vi "PQbuildConnectionString.vi"() -> ()   [LabVIEW 2019, in "libpqutility64.lvlib"]
doc: "Set up connection parameters, test the connectionstring and store it named into file. See PostgreSQL c-lib dokumentation for further information."
uses:
  libpqutility64.lvlib
  libpqlv/libpqlv.lvlib
  <vilib>/Utility/config.llb/NI_LVConfig.lvlib
  <vilib>/Utility/config.llb/Write Key (String).vi
panel:
  in  "Dateiname":string
  in  "Stopp":bool
  in  "Verbindungsname":string
  out "PQerrorMessage":string
  out "PQStatus":T1(ring)
  out "PQprotocolVersion":u32
  in  "Verbindung_testen":bool
  in  "Verbindung speichern":bool
  out "conninfo":string="\n"
  in  "requiressl":string
  in  "tty":string
  in  "options":string
  in  "connect_timeout":string
  in  "password":string
  in  "user":string
  in  "dbname":string
  in  "port":string
  in  "hostaddr":string
  in  "host":string
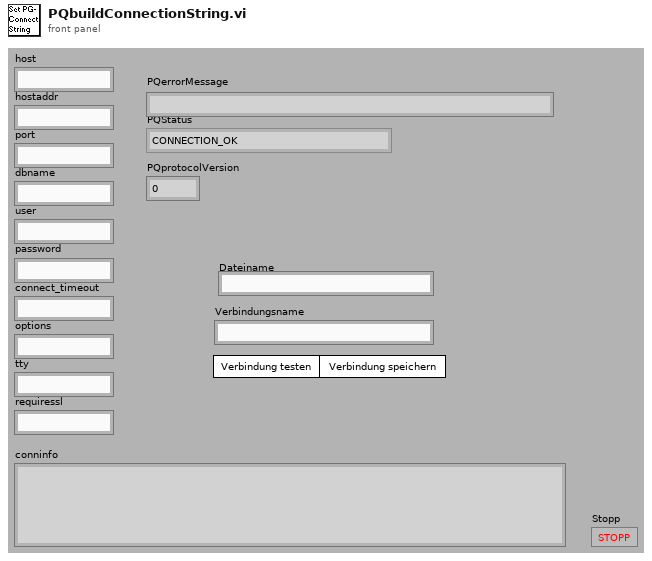
[diagram p1: front panel]
types:
  T1 = enum16{"CONNECTION_OK", "CONNECTION_BAD", "CONNECTION_STARTED", "CONNECTION_MADE", "CONNECTION_AWAITING_RESPONSE", "CONNECTION_AUTH_OK", "CONNECTION_SETENV", "CONNECTION_SSL_STARTUP", "CONNECTION_NEEDED"}
  T2 = enum32{"CONNECTION_OK", "CONNECTION_BAD", "CONNECTION_STARTED", "CONNECTION_MADE", "CONNECTION_AWAITING_RESPONSE", "CONNECTION_AUTH_OK", "CONNECTION_SETENV", "CONNECTION_SSL_STARTUP", "CONNECTION_NEEDED"}
  T3 = typedef "NI_LVConfig.lvlib/Config Data RefNum.ctl" = refnum<k1>
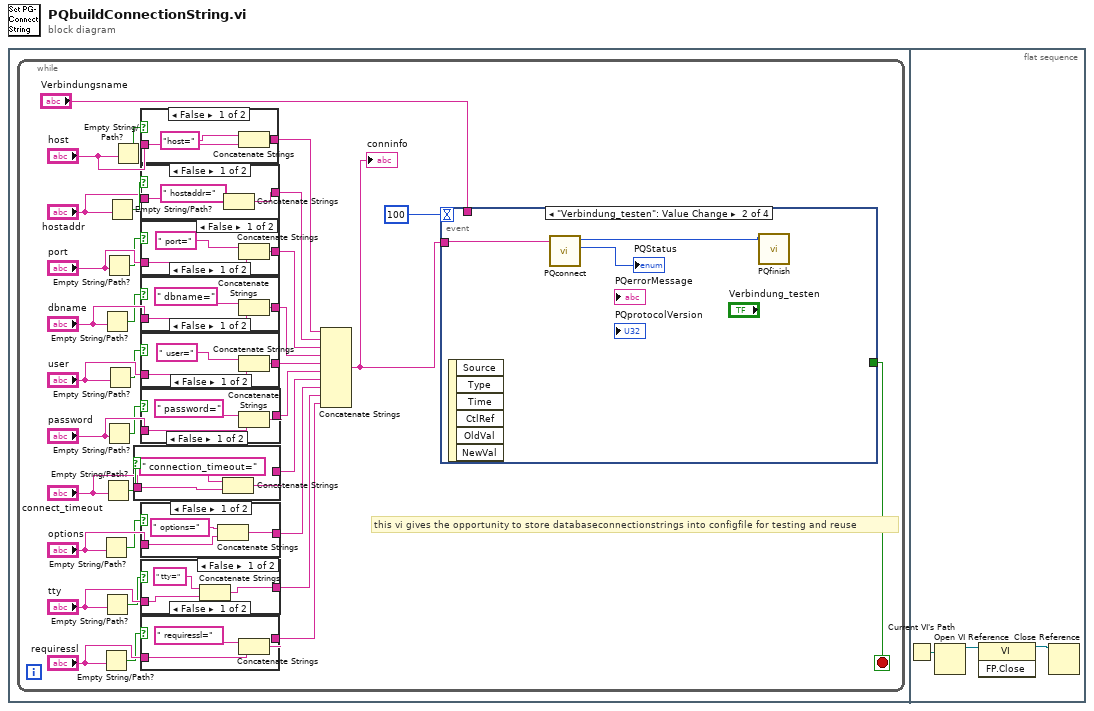
[diagram p0: block diagram]
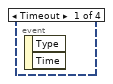
[diagram p2: hidden frame]
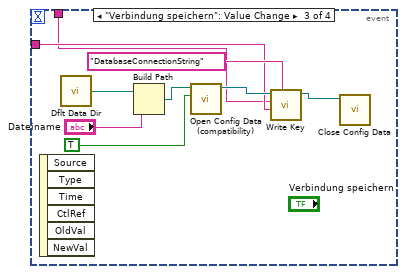
[diagram p3: hidden frame]
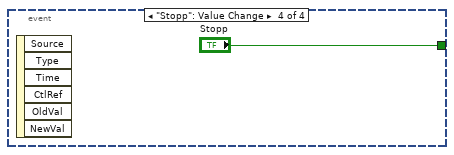
[diagram p4: hidden frame]
diagram:
  n1 = flat-sequence {
    frame #0 {
      n2 = while {
        stop <- w1 stop-if-true
        # "this vi gives the opportunity to store databaseconnectionstrings into configfile for testing and reuse"
        n3 = Empty String/Path? ("Leerer String/Pfad?")(string/path="options") -> (empty?=w18:bool)
        n4 = Empty String/Path? ("Leerer String/Pfad?")(string/path="requiressl") -> (empty?=w16:bool)
        n5 = Empty String/Path? ("Leerer String/Pfad?")(string/path="dbname") -> (empty?=w22:bool)
        n6 = Empty String/Path? ("Leerer String/Pfad?")(string/path="tty") -> (empty?=w17:bool)
        n7 = Empty String/Path? ("Leerer String/Pfad?")(string/path="connect_timeout") -> (empty?=w19:bool)
        n8 = Empty String/Path? ("Leerer String/Pfad?")(string/path="port") -> (empty?=w23:bool)
        n9 = Empty String/Path? ("Leerer String/Pfad?")(string/path="password") -> (empty?=w20:bool)
        n10 = Empty String/Path? ("Leerer String/Pfad?")(string/path="user") -> (empty?=w21:bool)
        n11 = Empty String/Path? ("Leerer String/Pfad?")(string/path="hostaddr") -> (empty?=w32:bool)
        n12 = Empty String/Path? ("Leerer String/Pfad?")(string/path="host") -> (empty?=w34:bool)
        n13 = case "Case-Struktur" shown="False" w19 {
          tunnel: "connect_timeout" -> [w62 w63]
          tunnel: [w60 w63] -> w10
          frame False {
            n14 = Concatenate Strings ("Strings verknüpfen")(" connection_timeout=", w62) -> (w60:string)
          }
          frame True {
          }
        }
        n15 = case "Case-Struktur" shown="False" w34 {
          tunnel: "host" -> [w85 w87]
          tunnel: [w84 w87] -> w15
          frame False {
            n16 = Concatenate Strings ("Strings verknüpfen")("host=", w85) -> (w84:string)
          }
          frame True {
          }
        }
        n17 = case "Case-Struktur" shown="False" w32 {
          tunnel: "hostaddr" -> [w81 w83]
          tunnel: [w80 w83] -> w6
          frame False {
            n18 = Concatenate Strings ("Strings verknüpfen")(" hostaddr=", w81) -> (w80:string)
          }
          frame True {
          }
        }
        n19 = case "Case-Struktur" shown="False" w23 {
          tunnel: "port" -> [w78 w79]
          tunnel: [w76 w79] -> w14
          frame False {
            n20 = Concatenate Strings ("Strings verknüpfen")(" port=", w78) -> (w76:string)
          }
          frame True {
          }
        }
        n21 = case "Case-Struktur" shown="False" w22 {
          tunnel: "dbname" -> [w74 w75]
          tunnel: [w72 w75] -> w13
          frame False {
            n22 = Concatenate Strings ("Strings verknüpfen")(" dbname=", w74) -> (w72:string)
          }
          frame True {
          }
        }
        n23 = case "Case-Struktur" shown="False" w21 {
          tunnel: "user" -> [w70 w71]
          tunnel: [w68 w71] -> w12
          frame False {
            n24 = Concatenate Strings ("Strings verknüpfen")(" user=", w70) -> (w68:string)
          }
          frame True {
          }
        }
        n25 = case "Case-Struktur" shown="False" w20 {
          tunnel: "password" -> [w66 w67]
          tunnel: [w64 w67] -> w11
          frame False {
            n26 = Concatenate Strings ("Strings verknüpfen")(" password=", w66) -> (w64:string)
          }
          frame True {
          }
        }
        n27 = case "Case-Struktur" shown="False" w18 {
          tunnel: "options" -> [w56 w59]
          tunnel: [w58 w59] -> w9
          frame False {
            n28 = Concatenate Strings ("Strings verknüpfen")(" options=", w56) -> (w58:string)
          }
          frame True {
          }
        }
        n29 = case "Case-Struktur" shown="False" w17 {
          tunnel: "tty" -> [w52 w55]
          tunnel: [w54 w55] -> w8
          frame False {
            n30 = Concatenate Strings ("Strings verknüpfen")(" tty=", w52) -> (w54:string)
          }
          frame True {
          }
        }
        n31 = case "Case-Struktur" shown="False" w16 {
          tunnel: "requiressl" -> [w50 w51]
          tunnel: [w48 w51] -> w7
          frame False {
            n32 = Concatenate Strings ("Strings verknüpfen")(" requiressl=", w50) -> (w48:string)
          }
          frame True {
          }
        }
        n33 = Concatenate Strings ("Strings verknüpfen")(w15, w6, w14, w13, w12, w11, w10, w9, w8, w7) -> (w2:string)
        "conninfo" <- w2
        n34 = event "Ereignisstruktur" shown="[1] \"Verbindung_testen\": Value Change" {
          selector: _ -> [_ _ _ _]
          dyn-events: _ -> [_ _ _ _]
          timeout: 100 -> [_ _ _ _]
          tunnel: w2 -> [_ w36 w39 _]
          tunnel: "Verbindungsname" -> [_ _ w38 _]
          tunnel: [_ _ _ "Stopp"] -> w1
          event Timeout {
            n35 = event-data() -> ()  [unwired: 1 in, 2 out]
          }
          event "Verbindung_testen": Value Change {
            n36 = event-data ("Ereignisdaten-Knoten")() -> ()  [unwired: 1 in, 6 out]
            n37 = call "PQconnect.vi"("conninfo"=w36) -> ("PQStatus"=→"PQStatus":T2, "conn"=w35:u64)  [unwired: 8 in, 1 out]
            n38 = call "PQfinish.vi"("conn"=w35) -> ()  [unwired: 10 in, 1 out]
          }
          event "Verbindung speichern": Value Change {
            n39 = event-data ("Ereignisdaten-Knoten")() -> ()  [unwired: 1 in, 6 out]
            n40 = call <vilib>:"Dflt Data Dir.vi"() -> ("App:Default Data Directory"=w44:path)
            n41 = Build Path ("Pfad erstellen")(base path=w44, name or relative path="Dateiname") -> (appended path=w40:path)
            n42 = call <vilib>:"Open Config Data (compatibility).vi"("create file if necessary (T)"=TRUE ("create file if necessary? (T)"), "configuration file path"=w40) -> ("refnum"=w45:T3)  [unwired: 7 in, 2 out]
            n43 = call-poly <vilib>:"Write Key.vi"("section"="DatabaseConnectionString", "value"=w39, "key"=w38, "refnum"=w45) -> ("refnum out"=w41:T3)  [unwired: 5 in, 2 out]
            n44 = call <vilib>:"Close Config Data.vi"("refnum"=w41) -> ()  [unwired: 9 in, 2 out]
          }
          event "Stopp": Value Change {
            n45 = event-data ("Ereignisdaten-Knoten")() -> ()  [unwired: 1 in, 6 out]
          }
        }
      }
    }
    frame #1 {
      n46 = Current VI's Path() -> (path=w88:path)
      n47 = Open VI Reference(vi path=w88) -> (vi reference=w89:refnum<vi>)  [unwired: 5 in, 1 out]
      n48 = invoke class="VI" method="FP.Close"(reference=w89) -> (reference out=w90:refnum<vi>)  [unwired: 2 in, 2 out]
      n49 = Close Reference(reference=w90) -> ()  [unwired: 1 in, 1 out]
    }
  }
